vi "SetNloopEnable.vi"(8 "error in":errorcluster, 9 "Nloop enable":enum16{"off", "on"}(ring), 10 "Settings In":T1={"position"={"Value"=0.0, "Min"=0.0, "Max"=25.0, "StepSize"=0.01, "Tolerance"=0.001, "ValueActual"=0.0}, "lowspeed"={"Value"=1000.0, "Min"=1.0, "Max"=40000.0, "StepSize"=500.0, "Tolerance"=0.0, "ValueActual"=0.0}, "highspeed"={"Value"=50000.0, "Min"=1000.0, "Max"=6000000.0, "StepSize"=500.0, "Tolerance"=0.0, "ValueActual"=0.0}, "Simulation"=enum."off", "Home"=enum."HOME", "EnableMotor"=enum."off", "Jog"=enum."POS (+)", "Motor steps/mm"=7874.016, "Encoder steps/mm"=629.921, "Nloop enable"=enum."off", "HomingIndex"=enum."off", "Encoder position"={"Value"=0.0, "Min"=0.0, "Max"=25.0, "StepSize"=0.01, "Tolerance"=0.001, "ValueActual"=0.0}} {"Encoder steps/mm" format="%#.6g"; "Motor steps/mm" format="%#.6g"}, 11 "reference (in)":refnum<class "_Controller.lvclass">) -> (0 "error out":errorcluster, 2 "Settings out":T1={"position"={"Value"=0.0, "Min"=0.0, "Max"=25.0, "StepSize"=0.01, "Tolerance"=0.001, "ValueActual"=0.0}, "lowspeed"={"Value"=1000.0, "Min"=1.0, "Max"=40000.0, "StepSize"=500.0, "Tolerance"=0.0, "ValueActual"=0.0}, "highspeed"={"Value"=50000.0, "Min"=1000.0, "Max"=6000000.0, "StepSize"=500.0, "Tolerance"=0.0, "ValueActual"=0.0}, "Simulation"=enum."off", "Home"=enum."HOME", "EnableMotor"=enum."off", "Jog"=enum."POS (+)", "Motor steps/mm"=7874.016, "Encoder steps/mm"=629.921, "Nloop enable"=enum."off", "HomingIndex"=enum."off", "Encoder position"={"Value"=0.0, "Min"=0.0, "Max"=25.0, "StepSize"=0.01, "Tolerance"=0.001, "ValueActual"=0.0}} {"Encoder steps/mm" format="%#.6g"; "Motor steps/mm" format="%#.6g"}, 3 "reference (out)":refnum<class "_Controller.lvclass">)   [LabVIEW 2020]
uses:
  settingsArcus_TypDef.ctl
  source/Device Drivers/shared/numericVariable_TypeDef.ctl
  _Controller.lvclass
  source/Device Drivers/BaseDriver/BaseDriver.lvclass
  Newmark-NSC-A.lvclass
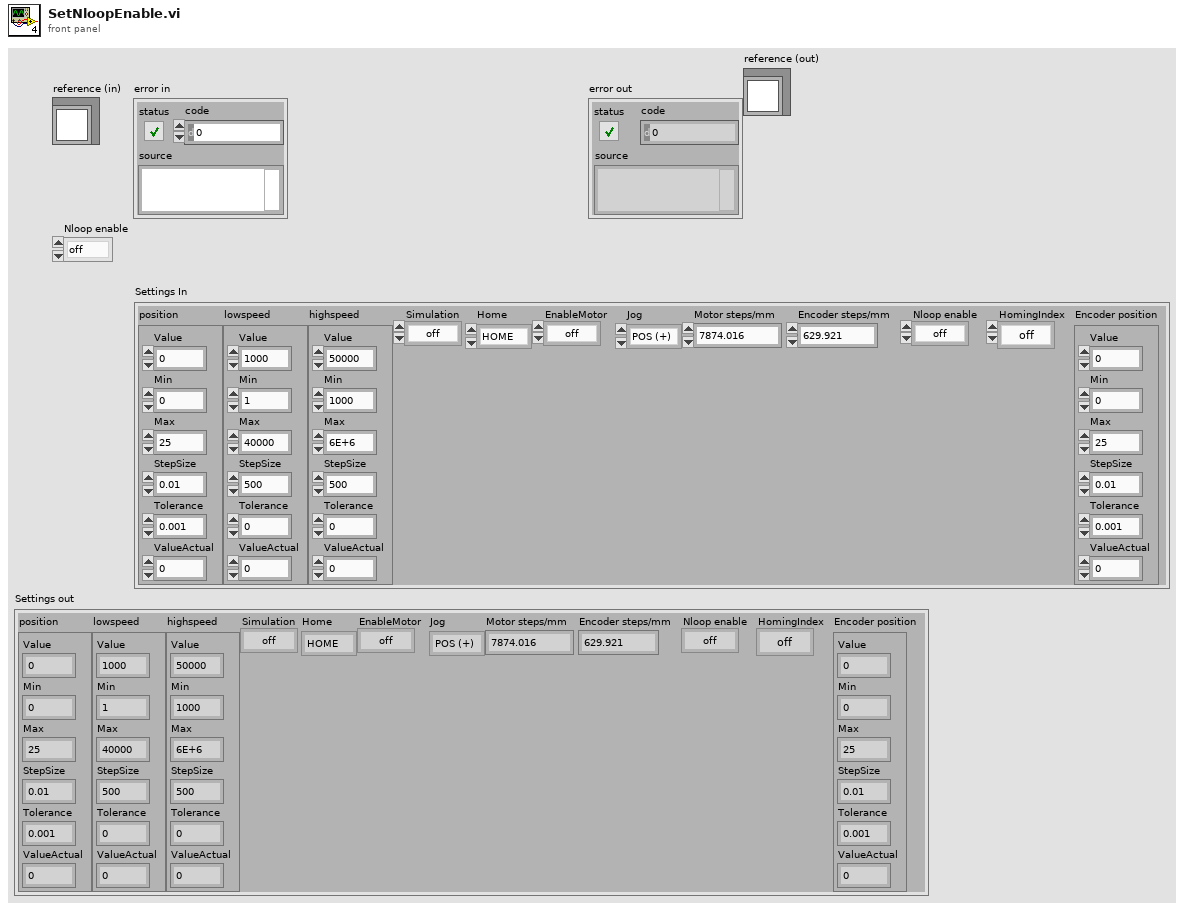
[diagram p1: front panel]
types:
  T1 = typedef "Newmark-NSC-A.lvclass/settingsArcus_TypDef.ctl" = cluster{"position":T2, "lowspeed":T2, "highspeed":T2, "Simulation":enum16{"off", "on"}, "Home":enum16{"HOME", "POS (+)", "NEG (-)", "done"}, "EnableMotor":enum16{"off", "on"}, "Jog":enum16{"POS (+)", "NEG (-)"}, "Motor steps/mm":dbl, "Encoder steps/mm":dbl, "Nloop enable":enum16{"off", "on"}, "HomingIndex":enum16{"off", "on"}, "Encoder position":T2}
  T2 = typedef "BaseDriver.lvclass/numericVariable_TypeDef.ctl" = cluster{"Value":dbl, "Min":dbl, "Max":dbl, "StepSize":dbl, "Tolerance":dbl, "ValueActual":dbl}
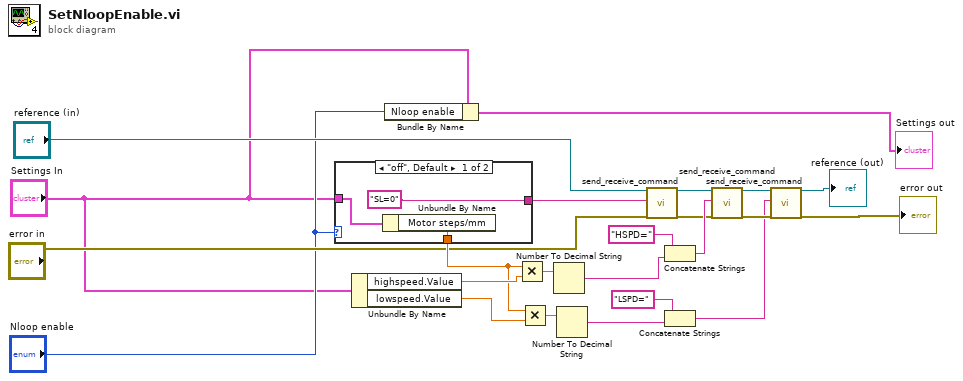
[diagram p0: block diagram]
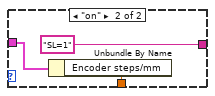
[diagram p2: hidden frame]
diagram:
  n1 = case shown="\"off\", Default" "Nloop enable" {
    tunnel: ["SL=0" "SL=1"] -> w23
    tunnel: "Settings In" -> [w25 w28]
    tunnel: [w24 w27] -> w13
    frame "off", Default {
      n2 = Unbundle By Name(w25) -> ("Motor steps/mm"=w24:dbl)
    }
    frame "on" {
      n3 = Unbundle By Name(w28) -> ("Encoder steps/mm"=w27:dbl)
    }
  }
  n4 = Unbundle By Name("Settings In") -> ("highspeed.Value"=w18:dbl, "lowspeed.Value"=w14:dbl)
  n5 = Bundle By Name(cluster="Settings In", "Nloop enable"="Nloop enable") -> (→"Settings out":T1)
  n6 = Multiply(x=w13, y=w18) -> (x*y=w21:dbl)
  n7 = Multiply(x=w13, y=w14) -> (x*y=w15:dbl)
  n8 = Number To Decimal String(number=w21) -> (decimal integer string=w22:string)  [unwired: 1 in]
  n9 = Number To Decimal String(number=w15) -> (decimal integer string=w11:string)  [unwired: 1 in]
  n10 = call "send_receive_command.vi"("reference (in)"="reference (in)", "ASCII Command (in)"=w23, "error in (no error)"="error in") -> ("reference (out)"=w17:refnum<class "_Controller.lvclass">, "error out"=w16:errorcluster)  [unwired: 12 in, 3 out]
  n11 = Concatenate Strings("HSPD=" ("write_string"), w22) -> (w20:string)
  n12 = Concatenate Strings("LSPD=" ("write_string"), w11) -> (w8:string)
  n13 = call "send_receive_command.vi"("reference (in)"=w17, "ASCII Command (in)"=w20, "error in (no error)"=w16) -> ("reference (out)"=w10:refnum<class "_Controller.lvclass">, "error out"=w9:errorcluster)  [unwired: 12 in, 3 out]
  n14 = call "send_receive_command.vi"("reference (in)"=w10, "ASCII Command (in)"=w8, "error in (no error)"=w9) -> ("reference (out)"=→"reference (out)":refnum<class "_Controller.lvclass">, "error out"=→"error out":errorcluster)  [unwired: 12 in, 3 out]
